vi "EX1.vi"() -> ()   [LabVIEW 2018]
panel:
  out "Division":dbl format="%#_3g"
  out "Multiplication":i32
  out "Soustraction":i32
  out "Addition":i32
  in  "b":i32 min=0 max=9
  in  "a":i32 min=0 max=9
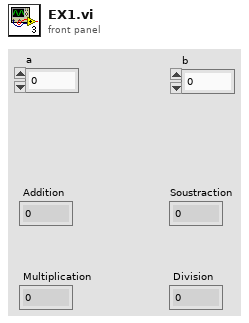
[diagram p1: front panel]
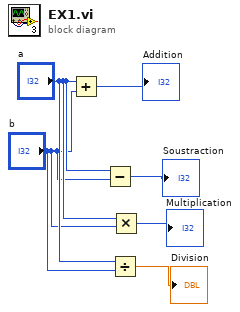
[diagram p0: block diagram]
diagram:
  n1 = Add(x="a", y="b") -> (x+y=→"Addition":i32)
  n2 = Subtract(x="a", y="b") -> (x-y=→"Soustraction":i32)
  n3 = Divide(x="a", y="b") -> (x/y=→"Division":dbl)
  n4 = Multiply(x="a", y="b") -> (x*y=→"Multiplication":i32)
